vi "svc_Integrate XY Data.vi"(10 "initial condition":dbl, 11 "XY":cluster{"X":dbl[], "Y":dbl[]}(graph)) -> (3 "integral(ydx)":dbl)   [LabVIEW 2017]
doc: "computes the integral of Y with respect to X\n\ncareful, this VI does not perform error checking and can return negative integral if positive function is integrated from right to left (this might even be useful if you are trying to find the area enclosed by a set of points)"
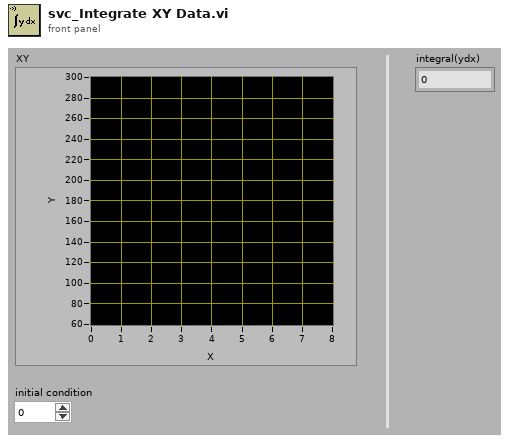
[diagram p1: front panel]
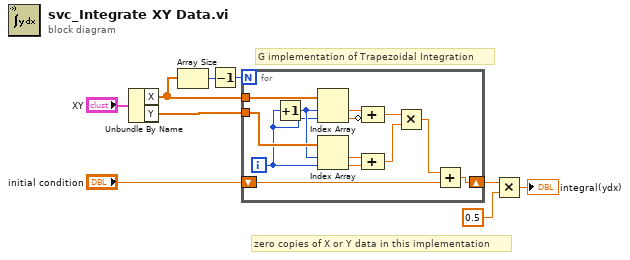
[diagram p0: block diagram]
diagram:
  # "zero copies of X or Y data in this implementation"
  # "G implementation of Trapezoidal Integration"
  n1 = Unbundle By Name("XY") -> ("X"=w7:dbl[], "Y"=w6:dbl[])
  n2 = Array Size(array=w7) -> (size(s)=w9:i32)
  n3 = Decrement(x=w9) -> (x-1=w8:i32)
  n4 = for {
    N: w8 -> [_]
    tunnel: w7 -> [w22]
    tunnel: w6 -> [w21]
    shift-right: [w12] -> w1
    shift-left: "initial condition" -> [w11]
    i -> [w19]
    n5 = Increment(x=w19) -> (x+1=w20:i32)
    n6 = Index Array(array=w22, index #1=w20, index #2=w19) -> (element #1=w17:dbl, element #2=w18:dbl)
    n7 = Index Array(array=w21, index #1=w20, index #2=w19) -> (element #1=w16:dbl, element #2=w15:dbl)
    n8 = Compound Arithmetic op=ADD(w17, invert w18) -> (w14:dbl)
    n9 = Compound Arithmetic op=ADD(w16, w15) -> (w13:dbl)
    n10 = Multiply(x=w14, y=w13) -> (x*y=w10:dbl)
    n11 = Add(x=w10, y=w11) -> (x+y=w12:dbl)
  }
  n12 = Multiply(x=w1, y=0.5) -> (x*y=→"integral(ydx)":dbl)
